vi "Serialisation Type.vi"(3 "JSONMessage in":refnum<class "WampMessage JSON.lvclass">) -> (1 "Serialisation Type":T1)   [LabVIEW 2020, in "wamplv.lvlib" / "WampMessage JSON.lvclass"]
uses:
  WampMessage JSON.lvclass
  WAMP Client/API/TypeDefs/Serialisation.ctl
  WampMessage JSON.lvclass/WampMessage JSON.ctl
  WAMP Client/WAMP Client.lvclass
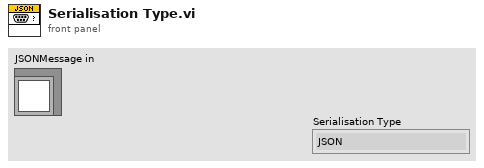
[diagram p1: front panel]
types:
  T1 = typedef "wamplv.lvlib/WAMP Client.lvclass/Serialisation.ctl" = enum16{"JSON", "MessagePack"}
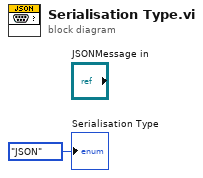
[diagram p0: block diagram]
diagram:
  "Serialisation Type" <- Serialisation."JSON" ("Serialisation Type")
